vi "FRAS CdG Reference.vi"(0 "Cluster DATA TCL-TCL":T1={"SF_Mode"=enum."Repos", "SF_8x1_donnees(t)"=[], "SF_dark_monopixels"=[], "SF_lambdas"=[0.0, 0.0], "SF_matrice_ABCD"=[[0.0, 0.0, 0.0, 0.0], [0.0, 0.0, 0.0, 0.0], [0.0, 0.0, 0.0, 0.0], [0.0, 0.0, 0.0, 0.0], [0.0, 0.0, 0.0, 0.0], [0.0, 0.0, 0.0, 0.0], [0.0, 0.0, 0.0, 0.0], [0.0, 0.0, 0.0, 0.0]], "SF_ref"=0.0, "SF_ref_mode"=enum."Repos", "SF_ref_fichier"=0.0, "SF_OPD_estime"=[0.0, 0.0], "SF_OPD_mesure"=[[0.0, 0.0]], "SF_OPD_residus"=[[0.0, 0.0]], "SF_OPD_commande"=0.0, "SF_Intensites"=[0.0, 0.0], "SF_variables"=[], "SF_gain_int"=0.0, "FRAS_Mode"=enum."Repos", "FRAS_image_a"=[], "FRAS_image_b"=[], "FRAS_ref_images"=[], "FRAS_ref_mode"=enum."Repos", "FRAS_ref_fichier"=[], "FRAS_taille_images"=0, "FRAS_pourcentage_seuil"=0.0, "FRAS_CdG_calibration"=FALSE, "FRAS_CdG(t)"=[], "FRAS_CdG(t+1)"=[], "FRAS_CdG_residus"=[], "FRAS_gain_int"=0.0, "PERT_Mode"=enum."Repos", "PERT_saut_frange"=0, "PERT_offset"=[0.0, 0.0], "PERT_rep_PI"=0.0, "Nb Repetitions"=32, "PERT_booléens"=[], "coefficients"=[], "matrice_commande"=[], "Commande"=[], "Stop"=FALSE, "Nb boucles"=0, "Nb Retards"=0, "Nb Echantillons"=32, "Sauvegarde"=FALSE, "Nb Echantillons Cam"=32, "Increment Dark"=32, "SF_v_mesure"=[0.0, 0.0], "NbRepetConsig"=0, "DimConsignExt"=0, "ConsignExt"=[], "SF_Ref'"=0.0, "FRAS_Ref'"=[]}, 7 "CdG(t)":dbl[](array[numeric])) -> (4 "Cluster DATA TCL-TCL":T1={"SF_Mode"=enum."Repos", "SF_8x1_donnees(t)"=[], "SF_dark_monopixels"=[], "SF_lambdas"=[0.0, 0.0], "SF_matrice_ABCD"=[[0.0, 0.0, 0.0, 0.0], [0.0, 0.0, 0.0, 0.0], [0.0, 0.0, 0.0, 0.0], [0.0, 0.0, 0.0, 0.0], [0.0, 0.0, 0.0, 0.0], [0.0, 0.0, 0.0, 0.0], [0.0, 0.0, 0.0, 0.0], [0.0, 0.0, 0.0, 0.0]], "SF_ref"=0.0, "SF_ref_mode"=enum."Repos", "SF_ref_fichier"=0.0, "SF_OPD_estime"=[0.0, 0.0], "SF_OPD_mesure"=[[0.0, 0.0]], "SF_OPD_residus"=[[0.0, 0.0]], "SF_OPD_commande"=0.0, "SF_Intensites"=[0.0, 0.0], "SF_variables"=[], "SF_gain_int"=0.0, "FRAS_Mode"=enum."Repos", "FRAS_image_a"=[], "FRAS_image_b"=[], "FRAS_ref_images"=[], "FRAS_ref_mode"=enum."Repos", "FRAS_ref_fichier"=[], "FRAS_taille_images"=0, "FRAS_pourcentage_seuil"=0.0, "FRAS_CdG_calibration"=FALSE, "FRAS_CdG(t)"=[], "FRAS_CdG(t+1)"=[], "FRAS_CdG_residus"=[], "FRAS_gain_int"=0.0, "PERT_Mode"=enum."Repos", "PERT_saut_frange"=0, "PERT_offset"=[0.0, 0.0], "PERT_rep_PI"=0.0, "Nb Repetitions"=32, "PERT_booléens"=[], "coefficients"=[], "matrice_commande"=[], "Commande"=[], "Stop"=FALSE, "Nb boucles"=0, "Nb Retards"=0, "Nb Echantillons"=32, "Sauvegarde"=FALSE, "Nb Echantillons Cam"=32, "Increment Dark"=32, "SF_v_mesure"=[0.0, 0.0], "NbRepetConsig"=0, "DimConsignExt"=0, "ConsignExt"=[], "SF_Ref'"=0.0, "FRAS_Ref'"=[]}, 8 "CdG res":dbl[](array[numeric]))   [LabVIEW 2020]
uses:
  DATACluster.ctl
panel:
  out "Refernece":dbl[](array[numeric])
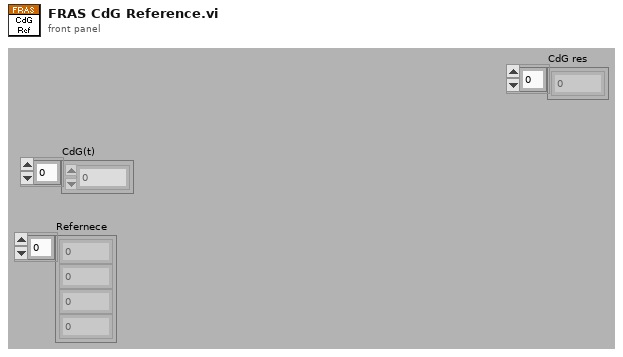
[diagram p1: front panel]
types:
  T1 = typedef "DATACluster.ctl" = cluster{"SF_Mode":enum16{"Repos", "Détection", "Acquisition", "Poursuite PID", "Poursuite Kalman", "Poursuite + contrôle"}, "SF_8x1_donnees(t)":dbl[], "SF_dark_monopixels":dbl[], "SF_lambdas":dbl[], "SF_matrice_ABCD":dbl[][], "SF_ref":dbl, "SF_ref_mode":enum16{"Repos", "Calibration", "Fichier"}, "SF_ref_fichier":dbl, "SF_OPD_estime":dbl[], "SF_OPD_mesure":dbl[][], "SF_OPD_residus":dbl[][], "SF_OPD_commande":dbl, "SF_Intensites":dbl[], "SF_variables":dbl[], "SF_gain_int":dbl, "FRAS_Mode":enum16{"Repos", "Détection", "Acquisition", "Poursuite", "Poursuite en a", "Poursuite en b"}, "FRAS_image_a":sgl[][], "FRAS_image_b":sgl[][], "FRAS_ref_images":sgl[][], "FRAS_ref_mode":enum16{"Repos", "Calibration", "Fichier"}, "FRAS_ref_fichier":sgl[][], "FRAS_taille_images":i32, "FRAS_pourcentage_seuil":sgl, "FRAS_CdG_calibration":bool, "FRAS_CdG(t)":dbl[], "FRAS_CdG(t+1)":dbl[], "FRAS_CdG_residus":dbl[], "FRAS_gain_int":dbl, "PERT_Mode":enum16{"Repos", "Calibration", "Fichier"}, "PERT_saut_frange":i8, "PERT_offset":dbl[], "PERT_rep_PI":dbl, "Nb Repetitions":i32, "PERT_booléens":bool[], "coefficients":dbl[], "matrice_commande":dbl[][], "Commande":dbl[][], "Stop":bool, "Nb boucles":i32, "Nb Retards":i16, "Nb Echantillons":i32, "Sauvegarde":bool, "Nb Echantillons Cam":i32, "Increment Dark":i32, "SF_v_mesure":dbl[], "NbRepetConsig":i32, "DimConsignExt":i32, "ConsignExt":dbl[][], "SF_Ref'":dbl, "FRAS_Ref'":dbl[][]}
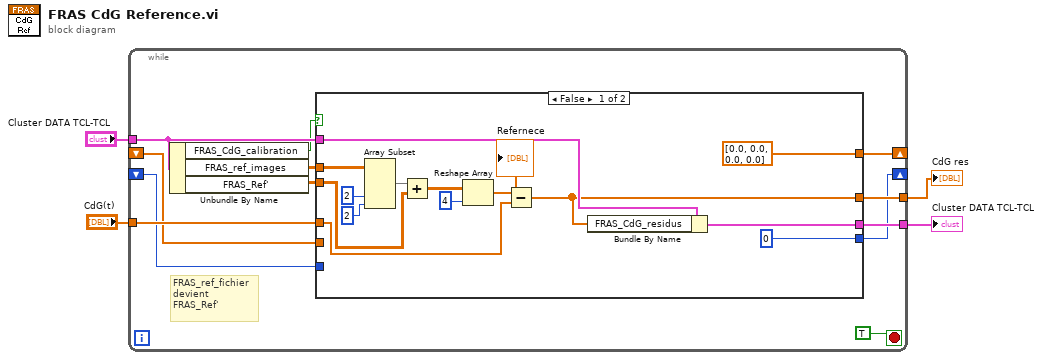
[diagram p0: block diagram]
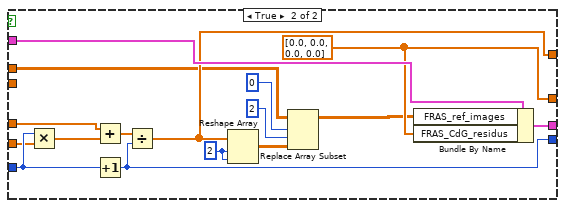
[diagram p2: hidden frame]
diagram:
  n1 = while {
    tunnel: [w16] -> w4
    tunnel: [w15] -> w3
    tunnel: "Cluster DATA TCL-TCL" -> [w14]
    tunnel: "CdG(t)" -> [w10]
    shift-right: [w9] -> _
    shift-left: _ -> [w8]
    shift-right: [w7] -> _
    shift-left: _ -> [w6]
    stop <- TRUE stop-if-true
    # "FRAS_ref_fichier\ndevient \nFRAS_Ref'"
    n2 = Unbundle By Name(w14) -> ("FRAS_CdG_calibration"=w13:bool, "FRAS_ref_images"=w12:sgl[][], "FRAS_Ref'"=w5:dbl[][])
    n3 = case shown="False" w13 {
      tunnel: [w28 w44] -> w15
      tunnel: w10 -> [w27 w39]
      tunnel: w14 -> [w30 w46]
      tunnel: [w29 w45] -> w16
      tunnel: w12 -> [w20 w35]
      tunnel: [0 w38] -> w9
      tunnel: w8 -> [_ w43]
      tunnel: [dbl[] [0.0, 0.0, 0.0, 0.0] w37] -> w7
      tunnel: w6 -> [_ w42]
      tunnel: w5 -> [w17 _]
      frame False {
        n4 = Array Subset(array=w20, index (col)=2 ("indice"), length (col)=2 ("longueur")) -> (w18:sgl[][])  [unwired: 2 in]
        n5 = Add(x=w18, y=w17) -> (x+y=w19:dbl[][])
        n6 = Reshape Array(w19, 4 ("taille de la dimension")) -> (w22:dbl[])
        "Refernece" <- w22
        n7 = Subtract(x=w22, y=w27) -> (x-y=w28:dbl[])
        n8 = Bundle By Name(cluster=w30, "FRAS_CdG_residus"=w28) -> (w29:T1)
      }
      frame True {
        w36 = 2 ("taille de la dimension")
        w44 = dbl[] [0.0, 0.0, 0.0, 0.0]
        n9 = Multiply(x=w43, y=w42) -> (x*y=w40:dbl[])
        n10 = Add(x=w39, y=w40) -> (x+y=w41:dbl[])
        n11 = Increment(x=w43) -> (x+1=w38:i32)
        n12 = Divide(x=w41, y=w38) -> (x/y=w37:dbl[])
        n13 = Reshape Array(w37, w36, w36) -> (w33:dbl[][])
        n14 = Replace Array Subset(array=w35, new element=w33, index (row)=0 ("indice désactivé (ligne)"), index (col)=2 ("indice désactivé (col)")) -> (w31:sgl[][])
        n15 = Bundle By Name(cluster=w46, "FRAS_ref_images"=w31, "FRAS_CdG_residus"=w44) -> (w45:T1)
      }
    }
  }
  "Cluster DATA TCL-TCL" <- w4
  "CdG res" <- w3
